vi "Read_Data_All_Fusing.vi"(7 "gain":dbl format="%#_6f", 9 "Center Frequency [Hz]":dbl=1000000000.0 format="%#.3p", 10 "Samples per read":i32=64000 format="%#.6g", 11 "path":path) -> (0 "error out":errorcluster)   [LabVIEW 2016]
uses:
  <instrlib>/niRFSG/niRFSG.llb/niRFSG Write Arb Waveform (I-Q).vi
panel:
  out "x = y?":bool
  out "Array Q (reshaped submatrix Q)":dbl[](array[numeric])
  out "Array I (reshaped submatrix I)":dbl[](array[numeric])
  out "submatrix Q":dbl[][](array[numeric])
  out "submatrix I":dbl[][](array[numeric])
  out "Waveform Graph Q":dbl[](graph)
  out "output array":dbl[][](array[numeric])
  out "Waveform Graph I":dbl[](graph)
  out "Samples Written":dbl format="%#.6g"
  in  "Direct Download":i32(ring)=1 items=["Disable", "Enable"]
  in  "Pre-filter Gain (dB)":dbl=-10.0 format="%_3f"
  in  "Power Level [dBm]":dbl=-20.0 format="%_3f"
  in  "IQ Rate (S/s)":dbl=25000000.0 format="%#.3p"
  in  "Signal Bandwidth":dbl=25000000.0 format="%#.3p"
  in  "Power Level Type":i32(ring)=7001 items=["Average Power"=7000, "Peak Power"=7001]
  out "Total Number Of Samples":dbl format="%#.6g"
  out "Actual IQ Rate (S/s)":dbl=8333333.333333333 format="%#.3p"
  in  "Tab Control":enum32{"Page 1"}(tab)
  out "element":i16
  in  "Stop":bool
  out "Generating":bool
  out "Progress Bar":dbl(slide) scale=0.0..100.0
  # "Setup Input"
  # "Runtime Output"
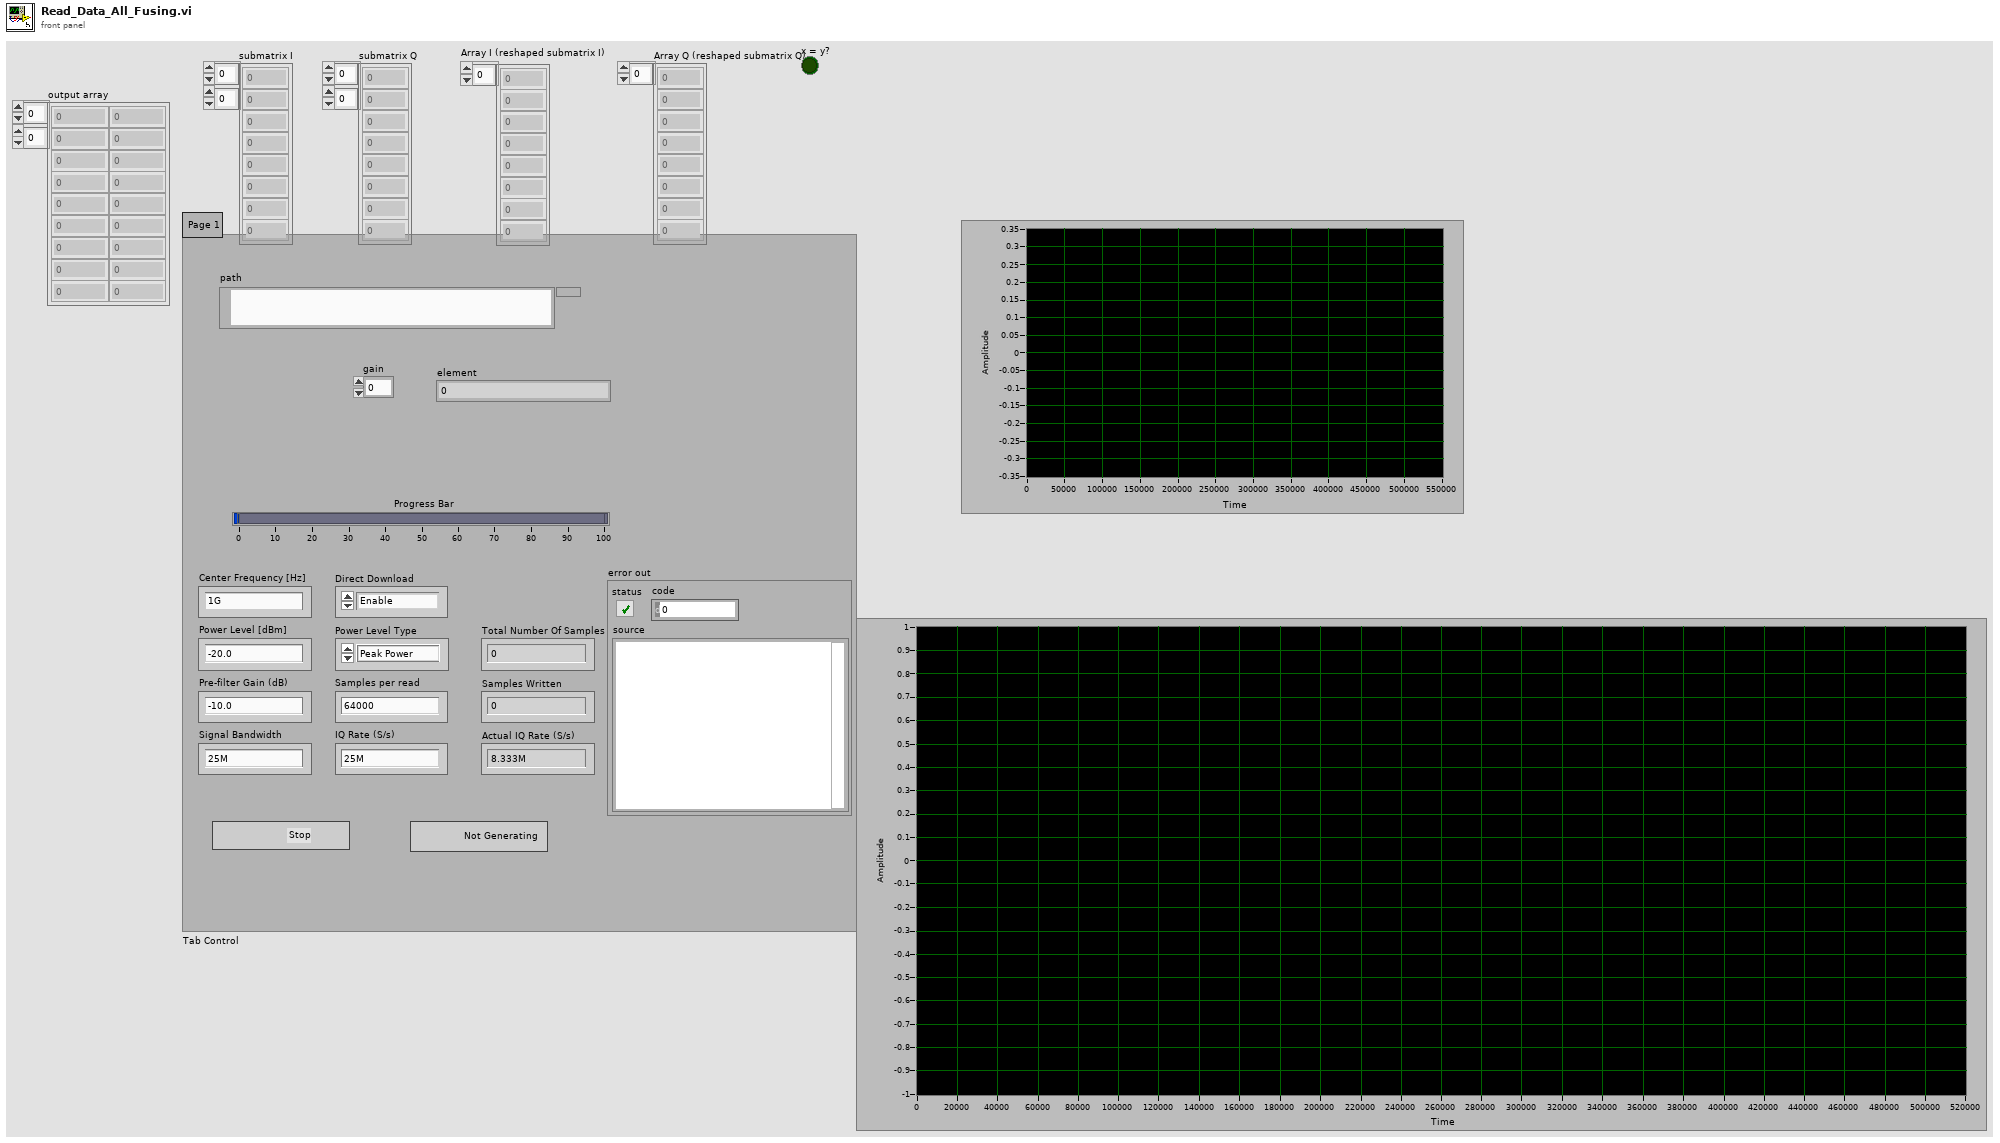
[diagram p1: front panel]
types:
  T1 = enum16{"big-endian, network order", "native, host order", "little-endian"}
  T2 = enum16{"open", "replace", "create", "open or create", "replace or create", "replace or create with confirmation"}
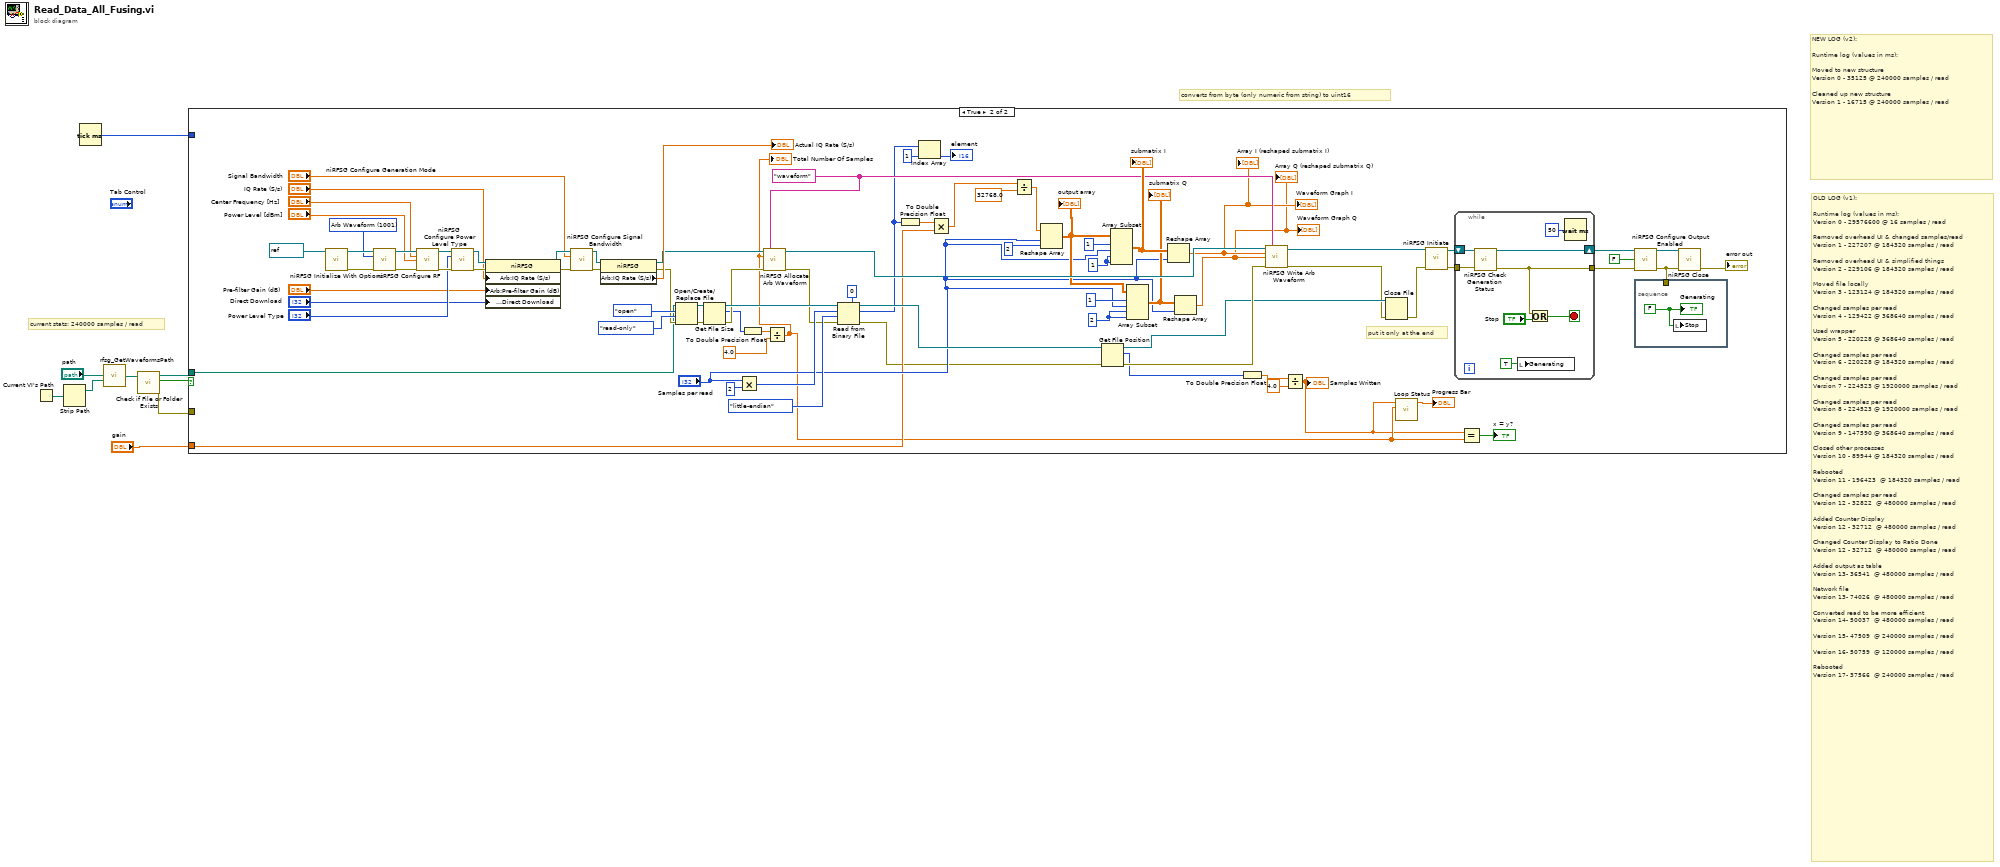
[diagram p0: block diagram]
diagram:
  # "NEW LOG (v2):\n\nRuntime log (values in ms):\n\nMoved to new structure\nVersion 0 - 35125 @ 240000 samples / read\n\nCleaned up new structure\nVersion 1 - 16715 @ 240000 samples / read"
  # "current stats: 240000 samples / read"
  # "OLD LOG (v1):\n\nRuntime log (values in ms):\nVersion 0 - 29576600 @ 16 samples / read\n\nRemoved overhead UI & changed samples/read\nVersion 1 - 227207 @ 184320 samples / read\n\nRemoved overhead UI & simplified things \nVersion 2 - 229106 @ 184320 samples / read\n\nMoved file locally\nVersion 3 - 123124 @ 184320 samples / read\n\nChanged samples per read\nVersion 4 - 129422 @ 368640 samples / read\n\nUsed wrapper\nVersion 5 - 220228 @ 368640 samples / read\n\nChanged samples per read\nVersion 6 - 220228 @ 184320 samples / read\n\nChanged samples per read\nVersion 7 - 224523 @ 1920000 samples / read\n\nChanged samples per read\nVersion 8 - 224523 @ 1920000 samples / read\n\nChanged samples per read\nVersion 9 - 147590 @ 368640 samples / read\n\nClosed other processes\nVersion 10 - 89944 @ 184320 samples / read\n\nRebooted\nVersion 11 - 196423  @ 184320 samples / read\n\nChanged samples per read\nVersion 12 - 32822  @ 480000 samples / read\n\nAdded Counter Display\nVersion 12 - 32712  @ 480000 samples / read\n\nChanged Counter Display to Ratio Done\nVersion 12 - 32712  @ 480000 samples / read\n\nAdded output as table\nVersion 13- 36541  @ 480000 samples / read\n\nNetwork file\nVersion 13- 74026  @ 480000 samples / read\n\nConverted read to be more efficient\nVersion 14- 50037  @ 480000 samples / read\n\nVersion 15- 47509  @ 240000 samples / read\n\nVersion 16- 50759  @ 120000 samples / read\n\nRebooted\nVersion 17- 37566  @ 240000 samples / read"
  # "converts from byte (only numeric from string) to uint16"
  n1 = Current VI's Path() -> (path=w3:path)
  n2 = Strip Path(path=w3) -> (stripped path=w4:path)  [unwired: 1 out]
  n3 = Tick Count (ms)() -> (millisecond timer value=w6:u32)
  n4 = call <instrlib>:"rfsg_GetWaveformsPath.vi"("wavefor file path (dialog if empty)"="path", "path relative to"=w4) -> ("waveforms path"=w2:path)  [unwired: 13 in]
  n5 = call <vilib>:"Check if File or Folder Exists.vi"("path"=w2) -> ("error out"=w7:errorcluster, "file or folder exists?"=w8:bool, "dup path"=w9:path)  [unwired: 8 in]
  n6 = case shown="True" w8 {
    tunnel: w9 -> [_ w21]
    tunnel: w7 -> [_ _]
    tunnel: w6 -> [_ _]
    tunnel: "gain" -> [_ w24]
    frame False {
    }
    frame True {
      w35 = 2 ("column 1")
      w37 = 1 ("column 1")
      w83 = 1001 items=["CW"=1000, "Arb Waveform"=1001, "Script"=1002] ("generation mode")
      w29 = "waveform" ("name")
      # "put it only at the end"
      n7 = call <instrlib>:"niRFSG Initialize With Options.vi"("resource name"=refnum<k15> "VST" ("Resource Name")) -> ("instrument handle"=w87:refnum<k15>, "error out"=w88:errorcluster)  [unwired: 13 in]
      n8 = call <instrlib>:"niRFSG Configure Generation Mode.vi"("instrument handle"=w87, "generation mode"=w83, "error in"=w88) -> ("instrument handle out"=w77:refnum<k15>, "error out"=w76:errorcluster)  [unwired: 11 in]
      n9 = call <instrlib>:"niRFSG Configure RF.vi"("instrument handle"=w77, "frequency (Hz)"="Center Frequency [Hz]", "power level (dBm)"="Power Level [dBm]", "error in"=w76) -> ("instrument handle out"=w70:refnum<k15>, "error out"=w68:errorcluster)  [unwired: 10 in]
      n10 = call <instrlib>:"niRFSG Configure Power Level Type.vi"("instrument handle"=w70, "power level type"="Power Level Type", "error in"=w68) -> ("instrument handle out"=w69:refnum<k15>, "error out"=w67:errorcluster)  [unwired: 11 in]
      n11 = property on="Property Node" class="niRFSG"(reference=w69, error in=w67, "Arb:IQ Rate (S/s)"="IQ Rate (S/s)", "Arb:Pre-filter Gain (dB)"="Pre-filter Gain (dB)", "Arb:Data Transfer:Direct Download"="Direct Download") -> (reference out=w71:refnum<k15>, error out=w60:errorcluster)
      n12 = call <instrlib>:"niRFSG Configure Signal Bandwidth.vi"("instrument handle"=w71, "signal bandwidth (Hz)"="Signal Bandwidth", "error in"=w60) -> ("instrument handle out"=w59:refnum<k15>, "error out"=w57:errorcluster)  [unwired: 11 in]
      n13 = property class="niRFSG"(reference=w59, error in=w57) -> (reference out=w58:refnum<k15>, error out=w56:errorcluster, "Arb:IQ Rate (S/s)"=→"Actual IQ Rate (S/s)":dbl)
      n14 = Open/Create/Replace File(file path (use dialog)=w21, error in=w56, operation (0:open)=T2."open", access (0:read/write)=enum16{"read/write", "read-only", "write-only"}."read-only") -> (refnum out=w63:refnum<file>, error out=w64:errorcluster)  [unwired: 2 in, 1 out]
      n15 = Get File Size(file=w63, error in=w64) -> (refnum out=w62:refnum<file>, size (in bytes)=w19:i64, 0:w55:errorcluster)
      n16 = Multiply(x="Samples per read", y=2) -> (x*y=w72:i32)
      n17 = To Double Precision Float(number=w19) -> (double precision float=w20:dbl)
      n18 = Divide(x=w20, y=4.0) -> (x/y=w12:dbl)
      "Total Number Of Samples" <- w12
      n19 = call <instrlib>:"niRFSG Allocate Arb Waveform.vi"("instrument handle"=w58, "name"=w29, "size in samples"=w12, "error in"=w55) -> ("instrument handle out"=w84:refnum<k15>, "error out"=w45:errorcluster)  [unwired: 10 in]
      n20 = Read from Binary File(5:i16 0 ("I16"), 8:w45, 9:T1."little-endian" ("byte order (0:big-endian, network order)"), 10:w72, 11:w62) -> (0:w18:errorcluster, 2:w28:i16[], 3:w40:refnum<file>)  [unwired: 1 in, 1 out]
      n21 = To Double Precision Float(number=w28) -> (double precision float=w23:dbl[])
      n22 = Index Array(array=w28, index=1) -> (element=→"element":i16)
      n23 = Multiply ("Multiply.vi")(x=w23, y=w24) -> (x*y=w31:dbl[])
      n24 = Divide(x=w31, y=32768.0) -> (x/y=w32:dbl[])
      n25 = Reshape Array(w32, "Samples per read", 2 ("dimension size")) -> (w30:dbl[][])
      "output array" <- w30
      n26 = Get File Position(4:w18, 7:w40) -> (0:w89:errorcluster, 2:w14:i64, 3:w75:refnum<file>)
      n27 = Array Subset(array=w30, index (row)=1 ("row 1"), length (row)="Samples per read", index (col)=w37, length (col)=w37) -> (w34:dbl[][])
      "submatrix I" <- w34
      n28 = Array Subset(array=w30, index (row)=1 ("row 1"), length (row)="Samples per read", index (col)=w35, length (col)=w35) -> (w33:dbl[][])
      "submatrix Q" <- w33
      n29 = Reshape Array(w34, "Samples per read") -> (w27:dbl[])
      "Waveform Graph I" <- w27
      "Array I (reshaped submatrix I)" <- w27
      n30 = Reshape Array(w33, "Samples per read") -> (w26:dbl[])
      "Waveform Graph Q" <- w26
      "Array Q (reshaped submatrix Q)" <- w26
      n31 = To Double Precision Float(number=w14) -> (double precision float=w41:dbl)
      n32 = call-poly <instrlib>:"niRFSG Write Arb Waveform.vi"("instrument handle"=w84, "name"=w29, "I Data"=w27, "Q Data"=w26, "error in"=w89) -> ("instrument handle out"=w82:refnum<k15>, "error out"=w46:errorcluster)  [unwired: 9 in]
      n33 = Divide(x=w41, y=4.0) -> (x/y=w11:dbl)
      "Samples Written" <- w11
      n34 = Close File(refnum=w75, error in=w46) -> (error out=w74:errorcluster)  [unwired: 1 out]
      n35 = call "Loop Status.vi"("total count"=w12, "current count"=w11) -> ("total count"=→"Progress Bar":dbl)  [unwired: 8 in, 1 out]
      n36 = call <instrlib>:"niRFSG Initiate.vi"("instrument handle"=w82, "error in"=w74) -> ("instrument handle out"=w81:refnum<k15>, "error out"=w47:errorcluster)  [unwired: 12 in]
      n37 = while {
        shift-right: [w99] -> w80
        shift-left: w81 -> [w100]
        tunnel: [w95] -> w48
        tunnel: w47 -> [w94]
        stop <- w93 stop-if-true
        n38 = call <instrlib>:"niRFSG Check Generation Status.vi"("instrument handle"=w100, "error in"=w94) -> ("instrument handle out"=w99:refnum<k15>, "error out"=w95:errorcluster)  [unwired: 11 in, 1 out]
        n39 = local write "Generating"(TRUE ("Boolean")) -> ()
        n40 = Or(x=w95, y="Stop") -> (x .or. y?=w93:bool)
        n41 = Wait (ms)(milliseconds to wait=u32 50) -> ()  [unwired: 1 out]
      }
      n42 = Equal?(x=w11, y=w12) -> (x = y?=→"x = y?":bool)
      n43 = call <instrlib>:"niRFSG Configure Output Enabled.vi"("instrument handle"=w80, "output enabled"=FALSE ("output enable"), "error in"=w48) -> ("instrument handle out"=w86:refnum<k15>, "error out"=w79:errorcluster)  [unwired: 11 in]
      n44 = stacked-sequence {
        tunnel: w79 -> [_]
        frame #0 {
          w92 = FALSE ("Boolean")
          n45 = local write "Stop"(w92) -> ()
          "Generating" <- w92
        }
      }
      n46 = call <instrlib>:"niRFSG Close.vi"("instrument handle"=w86, "error in"=w79) -> ("error out"=→"error out":errorcluster)  [unwired: 13 in]
    }
  }
